vi "Get Object Name.vi"(11 "Extracted Tokens":cluster{"token type":T1, T2}[](array[cluster])) -> (2 "found":bool, 3 "name":string)   [LabVIEW 2020, in "Multi Error Cluster.lvlib"]
uses:
  <vilib>/MultiError/TokenizeJSON/Multi Error Cluster.lvlib
  <vilib>/MultiError/TokenizeJSON/JSON Token Values.ctl
  <vilib>/MultiError/Errors Cluster Multiple Errors/JSON Token Descriptor.ctl
  <vilib>/MultiError/TokenizeJSON/JSON Raw Token Values.ctl
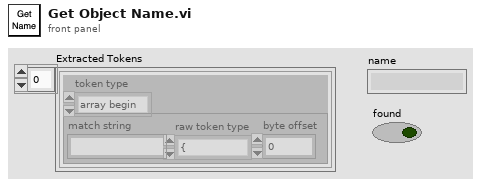
[diagram p1: front panel]
types:
  T1 = typedef "Multi Error Cluster.lvlib/JSON Token Values.ctl" = enum32{"array begin", "array end", "object begin", "object end", "value", "invalid", "name"}
  T2 = typedef "Multi Error Cluster.lvlib/JSON Token Descriptor.ctl" = cluster{"match string":string, "raw token type":T3, "byte offset ":i32}
  T3 = typedef "Multi Error Cluster.lvlib/JSON Raw Token Values.ctl" = enum32{"{", "}", "[", "]", ",", ":", "\"", "number", "string", "true", "false", "null", "invalid"}
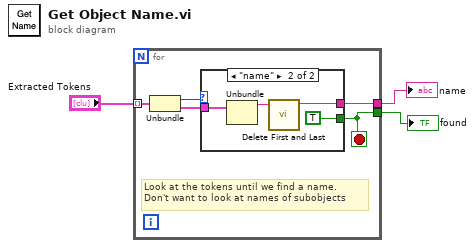
[diagram p0: block diagram]
diagram:
  n1 = for {
    tunnel: "Extracted Tokens" -> [w8] mode=indexing
    tunnel: [w5] -> w1
    tunnel: [w4] -> w2
    stop <- w4 stop-if-true
    # "Look at the tokens until we find a name.\nDon't want to look at names of subobjects"
    n2 = Unbundle(w8) -> ("token type"=w7:T1, w6:T2)
    n3 = case shown="\"name\"" w7 {
      tunnel: w6 -> [_ w12]
      tunnel: [_ w10] -> w5
      tunnel: [_ TRUE] -> w4
      frame Default {
      }
      frame "name" {
        n4 = Unbundle(w12) -> ("match string"=w11:string)  [unwired: 2 out]
        n5 = call <vilib>:"Delete First and Last.vi"("string in"=w11) -> ("string subset"=w10:string)  [unwired: 10 in]
      }
    }
  }
  "found" <- w2
  "name" <- w1
